vi "initalize dual gating(SubVI).vi"(0 "簇":T1={"initialize"=enum."SR830", "6221"={"6221 Resource"="GPIB0::24::INSTR", "Delta status"=FALSE, "电流|RMS(A)"=0.0}, "SR830+6221"={"source"=0, "Current(A)"=0.0, "阻抗(Ohm)"=0.0, "SR830 1"=FALSE, "SR830 2"=FALSE, "SR830 3"=FALSE, "SR830 4"=FALSE, "VISA 1"="", "VISA 2"="", "VISA 3"="", "VISA 4"="", "Reserve 1"=0, "Reserve 2"=-1, "Reserve 3"=-1, "Reserve 4"=-1, "Sensitivity 1"=-1, "Sensitivity 2"=-1, "Sensitivity 3"=-1, "Sensitivity 4"=-1, "量程入 1"=0, "量程入 2"=0, "量程入 3"=0, "量程入 4"=0}, "2400"={"2400"=FALSE, "VISA"="", "Output Level (0)"=1e-05, "Compliance  Level (0.1)"=10.0}, "ch"={"ch"=[], "current"=[], "change?"=[], "holding current\nwhen change ch?"=FALSE}, "Instrument"={"325 Resource "="GPIB0::13::INSTR", "Input (0:A) 325"=0, "Heater Output (1:1) 325"=1, "340 Resource"="GPIB0::14::INSTR", "Input (0:A) 340"=0, "Loop (0: 1)"=0, "Input (0:B) 340"=1, "Loop (1: 1)"=0, "340 Status"=refnum, "Instrument Type"=enum."PPMS-Rotate", "quantum design"=refnum, "semaphore 325"=refnum, "TCP master instance"=refnum, "M24C Resource"="GPIB0::24::INSTR", "4G supply"="GPIB0::24::INSTR", "Temp Status 24C"=refnum, "Temp"=refnum, "9T信号"=refnum, "limit"={"Field limit"=0.0, "Field rate limit"=0.0, "Temp limit"=0.0, "Temp low limit"=0.0, "Temp rate limit "=0.0}, "4g supply status"=refnum, "vi路径"="", "in-plane"="", "out-plane"="", "in-plane signal"=FALSE, "out-plane signal"=FALSE, "in plane 信号"=refnum, "pzt volt"=refnum, "Aborting"=refnum, "数据文件"=refnum, "warning"=refnum, "750 visa"="", "750 rotate"="", "335 Status 2"=refnum, "335 Resource "="GPIB0::24::INSTR", "Input (0:A) 335"=0, "Input (0:B) 335"=1, "Heater Output (1:1) 335"=1, "semaphore 340"=refnum, "semaphore 335"=refnum, "325 Status"=refnum, "semaphore 750"=refnum, "750 field status"=refnum, "camg 振荡状态"=refnum, "列表框"=refnum, "编辑列表框？"=refnum, "camg Rate"=refnum, "行数"=refnum}, "2614B"={"2614B chA"=FALSE, "2614B chB"=FALSE, "VISA"=""}, "33522b"={"33522b resource name"="GPIB0::16::INSTR", "零电压"=0.0, "最大电压"=148.0, "间隔"=4.0, "最小电压"=-48.0, "PZT Scan?"=FALSE}, "gating type"=enum."2614(daul)", "层数"=0, "行数"=0, "是否处理"=[]} {"Instrument"."Loop (1: 1)" items=["1"=1, "2"=2]; "Instrument"."Loop (0: 1)" items=["1"=1, "2"=2]; "Instrument"."Input (0:B) 340" items=["A", "B", "C", "D"]; "Instrument"."Heater Output (1:1) 335" items=["1"=1, "2"=2]; "Instrument"."Input (0:B) 335" items=["A", "B"]; "Instrument"."Input (0:A) 335" items=["A", "B"]; "Instrument"."Heater Output (1:1) 325" items=["1"=1, "2"=2]; "Instrument"."Input (0:A) 325" items=["A", "B"]; "Instrument"."Input (0:A) 340" items=["1"=1, "2"=2]; "SR830+6221"."Sensitivity 4" items=["量程每次测量会判定", "量程不变为设定值"]; "SR830+6221"."Sensitivity 3" items=["Auto Reserve"=-1, "High Reserve"=0, "Normal"=1, "Low Noise"=2]; "SR830+6221"."Sensitivity 1" items=["Auto Reserve"=-1, "High Reserve"=0, "Normal"=1, "Low Noise"=2]; "SR830+6221"."Sensitivity 2" items=["Auto Reserve"=-1, "High Reserve"=0, "Normal"=1, "Low Noise"=2]; "SR830+6221"."Reserve 4" items=["量程每次测量会判定", "量程不变为设定值"]; "SR830+6221"."Reserve 3" items=["Auto Reserve"=-1, "High Reserve"=0, "Normal"=1, "Low Noise"=2]; "SR830+6221"."Reserve 2" items=["Auto Reserve"=-1, "High Reserve"=0, "Normal"=1, "Low Noise"=2]; "SR830+6221"."Reserve 1" items=["Auto Reserve"=-1, "High Reserve"=0, "Normal"=1, "Low Noise"=2]; "SR830+6221"."source" items=["SR830 1", "SR830 2", "SR830 3", "SR830 4"]}, 2 "字符串":string) -> (7 "输出簇":T1={"initialize"=enum."SR830", "6221"={"6221 Resource"="GPIB0::24::INSTR", "Delta status"=FALSE, "电流|RMS(A)"=0.0}, "SR830+6221"={"source"=0, "Current(A)"=0.0, "阻抗(Ohm)"=0.0, "SR830 1"=FALSE, "SR830 2"=FALSE, "SR830 3"=FALSE, "SR830 4"=FALSE, "VISA 1"="", "VISA 2"="", "VISA 3"="", "VISA 4"="", "Reserve 1"=0, "Reserve 2"=-1, "Reserve 3"=-1, "Reserve 4"=-1, "Sensitivity 1"=-1, "Sensitivity 2"=-1, "Sensitivity 3"=-1, "Sensitivity 4"=-1, "量程入 1"=0, "量程入 2"=0, "量程入 3"=0, "量程入 4"=0}, "2400"={"2400"=FALSE, "VISA"="", "Output Level (0)"=1e-05, "Compliance  Level (0.1)"=10.0}, "ch"={"ch"=[], "current"=[], "change?"=[], "holding current\nwhen change ch?"=FALSE}, "Instrument"={"325 Resource "="GPIB0::13::INSTR", "Input (0:A) 325"=0, "Heater Output (1:1) 325"=1, "340 Resource"="GPIB0::14::INSTR", "Input (0:A) 340"=0, "Loop (0: 1)"=0, "Input (0:B) 340"=1, "Loop (1: 1)"=0, "340 Status"=refnum, "Instrument Type"=enum."PPMS-Rotate", "quantum design"=refnum, "semaphore 325"=refnum, "TCP master instance"=refnum, "M24C Resource"="GPIB0::24::INSTR", "4G supply"="GPIB0::24::INSTR", "Temp Status 24C"=refnum, "Temp"=refnum, "9T信号"=refnum, "limit"={"Field limit"=0.0, "Field rate limit"=0.0, "Temp limit"=0.0, "Temp low limit"=0.0, "Temp rate limit "=0.0}, "4g supply status"=refnum, "vi路径"="", "in-plane"="", "out-plane"="", "in-plane signal"=FALSE, "out-plane signal"=FALSE, "in plane 信号"=refnum, "pzt volt"=refnum, "Aborting"=refnum, "数据文件"=refnum, "warning"=refnum, "750 visa"="", "750 rotate"="", "335 Status 2"=refnum, "335 Resource "="GPIB0::24::INSTR", "Input (0:A) 335"=0, "Input (0:B) 335"=1, "Heater Output (1:1) 335"=1, "semaphore 340"=refnum, "semaphore 335"=refnum, "325 Status"=refnum, "semaphore 750"=refnum, "750 field status"=refnum, "camg 振荡状态"=refnum, "列表框"=refnum, "编辑列表框？"=refnum, "camg Rate"=refnum, "行数"=refnum}, "2614B"={"2614B chA"=FALSE, "2614B chB"=FALSE, "VISA"=""}, "33522b"={"33522b resource name"="GPIB0::16::INSTR", "零电压"=0.0, "最大电压"=148.0, "间隔"=4.0, "最小电压"=-48.0, "PZT Scan?"=FALSE}, "gating type"=enum."2614(daul)", "层数"=0, "行数"=0, "是否处理"=[]} {"Instrument"."Loop (1: 1)" items=["1"=1, "2"=2]; "Instrument"."Loop (0: 1)" items=["1"=1, "2"=2]; "Instrument"."Input (0:B) 340" items=["A", "B", "C", "D"]; "Instrument"."Heater Output (1:1) 335" items=["1"=1, "2"=2]; "Instrument"."Input (0:B) 335" items=["A", "B"]; "Instrument"."Input (0:A) 335" items=["A", "B"]; "Instrument"."Heater Output (1:1) 325" items=["1"=1, "2"=2]; "Instrument"."Input (0:A) 325" items=["A", "B"]; "Instrument"."Input (0:A) 340" items=["1"=1, "2"=2]; "SR830+6221"."Sensitivity 4" items=["量程每次测量会判定", "量程不变为设定值"]; "SR830+6221"."Sensitivity 3" items=["Auto Reserve"=-1, "High Reserve"=0, "Normal"=1, "Low Noise"=2]; "SR830+6221"."Sensitivity 1" items=["Auto Reserve"=-1, "High Reserve"=0, "Normal"=1, "Low Noise"=2]; "SR830+6221"."Sensitivity 2" items=["Auto Reserve"=-1, "High Reserve"=0, "Normal"=1, "Low Noise"=2]; "SR830+6221"."Reserve 4" items=["量程每次测量会判定", "量程不变为设定值"]; "SR830+6221"."Reserve 3" items=["Auto Reserve"=-1, "High Reserve"=0, "Normal"=1, "Low Noise"=2]; "SR830+6221"."Reserve 2" items=["Auto Reserve"=-1, "High Reserve"=0, "Normal"=1, "Low Noise"=2]; "SR830+6221"."Reserve 1" items=["Auto Reserve"=-1, "High Reserve"=0, "Normal"=1, "Low Noise"=2]; "SR830+6221"."source" items=["SR830 1", "SR830 2", "SR830 3", "SR830 4"]})   [LabVIEW 2019, in "initialize.lvlib"]
uses:
  initialize.lvlib
  ctl/config.ctl
  <vilib>/NI/Modbus Library/API/Master/Modbus Master.lvclass
  ctl/initialize.ctl
  ctl/Instrument.ctl
  ctl/335 state.ctl
  ctl/Instrument Type.ctl
  lib/QDInstrument.dll
  ctl/limit.ctl
  ctl/9T mag field stauts.ctl
  ctl/warning.ctl
  ctl/Gating type.ctl
  lib/Keithley 2600 Series/Public/Configure/Source/Configure Source (Range).vi
  lib/Keithley 2600 Series/Public/Configure/Source/Configure Source (Limit).vi
  lib/Keithley 2600 Series/Keithley 2600 Series.lvlib
panel:
  in  "Current Limit B (0.1 A) 2":dbl=0.1
  in  "Current Limit A (0.1 A)":dbl=0.1
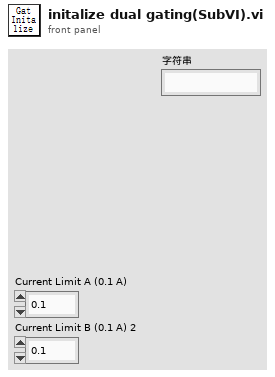
[diagram p1: front panel]
types:
  T1 = typedef "config.ctl" = cluster{"initialize":T2, "6221":cluster{"6221 Resource":refnum<visa-resource-name>, "Delta status":bool, "电流|RMS(A)":dbl}, "SR830+6221":cluster{"source":u16, "Current(A)":dbl, "阻抗(Ohm)":dbl, "SR830 1":bool, "SR830 2":bool, "SR830 3":bool, "SR830 4":bool, "VISA 1":refnum<visa-resource-name>, "VISA 2":refnum<visa-resource-name>, "VISA 3":refnum<visa-resource-name>, "VISA 4":refnum<visa-resource-name>, "Reserve 1":i16, "Reserve 2":i16, "Reserve 3":i16, "Reserve 4":i16, "Sensitivity 1":i16, "Sensitivity 2":i16, "Sensitivity 3":i16, "Sensitivity 4":i16, "量程入 1":i32, "量程入 2":i32, "量程入 3":i32, "量程入 4":i32}, "2400":cluster{"2400":bool, "VISA":refnum<visa-resource-name>, "Output Level (0)":dbl, "Compliance  Level (0.1)":dbl}, "ch":cluster{"ch":i32[], "current":dbl[], "change?":bool[], "holding current\nwhen change ch?":bool}, "Instrument":T3, "2614B":cluster{"2614B chA":bool, "2614B chB":bool, "VISA":refnum<visa-resource-name>}, "33522b":cluster{"33522b resource name":refnum<visa-resource-name>, "零电压":dbl, "最大电压":dbl, "间隔":dbl, "最小电压":dbl, "PZT Scan?":bool}, "gating type":T7, "层数":i32, "行数":i32, "是否处理":bool[]}
  T2 = typedef "initialize.ctl" = enum16{"SR830", "keithley6221-SR830", "Delta", "Delta-tunnelling", "keithley6221-2182-DC", "PZT", "4200"}
  T3 = typedef "Instrument.ctl" = cluster{"325 Resource ":refnum<visa-resource-name>, "Input (0:A) 325":u16, "Heater Output (1:1) 325":u16, "340 Resource":refnum<visa-resource-name>, "Input (0:A) 340":u16, "Loop (0: 1)":u16, "Input (0:B) 340":u16, "Loop (1: 1)":u16, "340 Status":refnum<vi>, "Instrument Type":T4, "quantum design":refnum<k24>, "semaphore 325":T5, "TCP master instance":refnum<class "Modbus Master.lvclass">, "M24C Resource":refnum<visa-resource-name>, "4G supply":refnum<visa-resource-name>, "Temp Status 24C":refnum<vi>, "Temp":refnum<vi>, "9T信号":T5, "limit":T6, "4g supply status":refnum<vi>, "vi路径":string, "in-plane":refnum<visa-resource-name>, "out-plane":refnum<visa-resource-name>, "in-plane signal":bool, "out-plane signal":bool, "in plane 信号":T5, "pzt volt":refnum<vi>, "Aborting":refnum<vi>, "数据文件":refnum<vi>, "warning":refnum<vi>, "750 visa":refnum<visa-resource-name>, "750 rotate":refnum<visa-resource-name>, "335 Status 2":refnum<vi>, "335 Resource ":refnum<visa-resource-name>, "Input (0:A) 335":u16, "Input (0:B) 335":u16, "Heater Output (1:1) 335":u16, "semaphore 340":T5, "semaphore 335":T5, "325 Status":refnum<vi>, "semaphore 750":T5, "750 field status":refnum<vi>, "camg 振荡状态":refnum<vi>, "列表框":refnum<vi>, "编辑列表框？":refnum<vi>, "camg Rate":refnum<vi>, "行数":refnum<vi>}
  T4 = typedef "Instrument Type.ctl" = enum16{"PPMS", "VersaLab", "DynaCool", "SVSM", "PPMS-Rotate", "Lakeshore335", "lengtou2", "9T mag", "9T cmag rotate", "test"}
  T5 = typedef "Semaphore RefNum" = refnum<k1>
  T6 = typedef "limit.ctl" = cluster{"Field limit":dbl, "Field rate limit":dbl, "Temp limit":dbl, "Temp low limit":dbl, "Temp rate limit ":dbl}
  T7 = typedef "Gating type.ctl" = enum32{"null", "2614(daul)", "2400"}
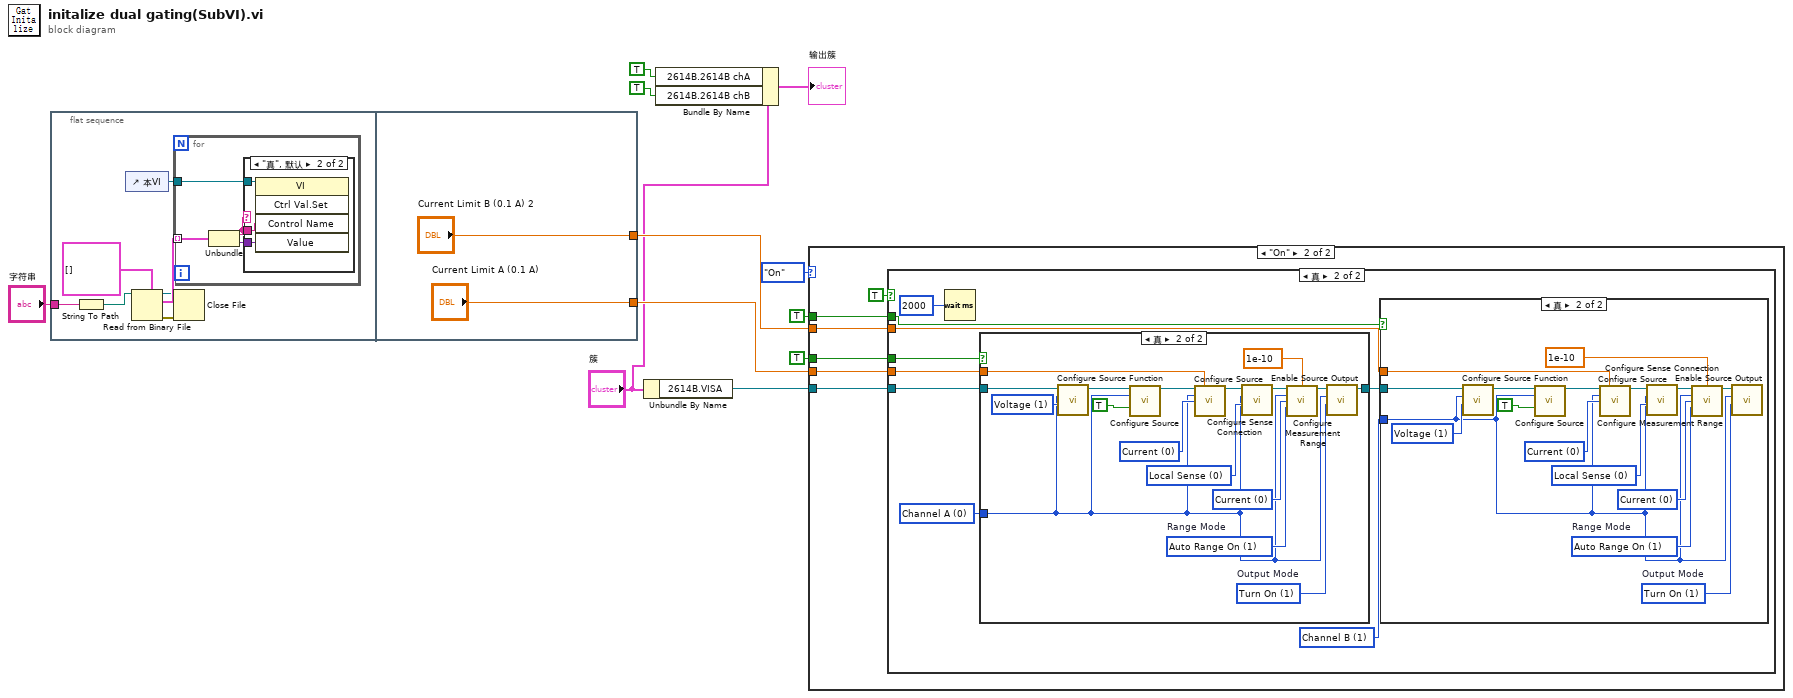
[diagram p0: block diagram]
diagram:
  n1 = flat-sequence {
    tunnel: "字符串" -> [w12]
    tunnel: ["Current Limit A (0.1 A)"] -> w8
    tunnel: ["Current Limit B (0.1 A) 2"] -> w9
    frame #0 {
      n2 = String To Path(string=w12) -> (path=w17:path)
      n3 = control-ref of="本VI"() -> (w18:refnum<vi>)
      n4 = Read from Binary File(5:cluster{"Name":string, "Variant Data":variant}[] [] ("控件值:获取全部"), 11:w17) -> (0:w13:errorcluster, 2:w15:cluster{"Name":string, "Variant Data":variant}[], 3:w14:refnum<file>)  [unwired: 4 in, 1 out]
      n5 = for {
        tunnel: w15 -> [w22] mode=indexing
        tunnel: w18 -> [w21]
        n6 = Unbundle(w22) -> ("Name"=w19:string, "Variant Data"=w20:variant)
        n7 = case shown="\"真\", 默认" w19 {
          tunnel: w21 -> [_ w25]
          tunnel: w19 -> [_ w24]
          tunnel: w20 -> [_ w23]
          frame "cancel", "load", "model", "ok" {
          }
          frame "真", Default {
            n8 = invoke class="VI" method="Ctrl Val.Set"(reference=w25, "Control Name"=w24, "Value"=w23) -> ()  [unwired: 2 in, 5 out]
          }
        }
      }
      n9 = Close File(refnum=w14, error in=w13) -> ()  [unwired: 2 out]
    }
    frame #1 {
    }
  }
  n10 = Unbundle By Name("簇") -> ("2614B.VISA"=w7:refnum<visa-resource-name>)
  n11 = Bundle By Name(cluster="簇", "2614B.2614B chA"=TRUE, "2614B.2614B chB"=TRUE) -> (→"输出簇":T1)
  n12 = case shown="\"On\"" enum16{"Off", "On"}."On" ("Output State") {
    tunnel: TRUE ("chB") -> [_ w32]
    tunnel: w9 -> [_ w31]
    tunnel: TRUE ("chA") -> [_ w30]
    tunnel: w7 -> [_ w29]
    tunnel: w8 -> [_ w28]
    frame "Off", Default {
    }
    frame "On" {
      n13 = case shown="真" TRUE {
        tunnel: w32 -> [_ w40]
        tunnel: w31 -> [_ w38]
        tunnel: w30 -> [_ w37]
        tunnel: w29 -> [_ w36]
        tunnel: w28 -> [_ w34]
        frame False {
        }
        frame True {
          w35 = 0 items=["Channel A", "Channel B"] ("Source Measure Unit Channel (0: Channel A)")
          w39 = 1 items=["Channel A", "Channel B"] ("Source Measure Unit Channel (0: Channel A)")
          n14 = Wait (ms)(milliseconds to wait=u32 2000) -> ()  [unwired: 1 out]
          n15 = case shown="真" w37 {
            tunnel: w36 -> [w59 w66]
            tunnel: w35 -> [_ w65]
            tunnel: w34 -> [_ w63]
            tunnel: [w59 w61] -> w41
            frame False {
            }
            frame True {
              w72 = 0 items=["Local Sense", "Remote Sense"] ("Sense Mode (0: Local Sense)")
              w71 = 0 items=["Current", "Voltage"] ("Range Type (0: Current)")
              w69 = 0 items=["Current", "Voltage", "Power"] ("Limit Type (1: Voltage)")
              w67 = 1 items=["Current", "Voltage"] ("Source Function (1: Voltage)")
              w70 = 1 items=["Auto Range Off", "Auto Range On", "Auto Range Follow Limit"]  # Range Mode
              w73 = 1 items=["Turn off", "Turn On", "High-Z"]  # Output Mode
              n16 = call "Configure Source Function.vi"("Source Function (1: Voltage)"=w67, "Source Measure Unit Channel (0: Channel A)"=w65, "VISA resource name"=w66) -> ("VISA resource name out"=w74:refnum<visa-resource-name>)  [unwired: 7 in, 1 out]
              n17 = call-poly "Configure Source.vi"("VISA resource name"=w74, "Source Measure Unit Channel (0: Channel A)"=w65, "Auto Range (T: Enable)"=TRUE) -> ("VISA resource name out"=w75:refnum<visa-resource-name>)  [unwired: 11 in, 1 out]
              n18 = call-poly "Configure Source.vi"("VISA resource name"=w75, "Current Limit (0.1 A)"=w63, "Source Measure Unit Channel (0: Channel A)"=w65, "Limit Type (1: Voltage)"=w69) -> ("VISA resource name out"=w76:refnum<visa-resource-name>)  [unwired: 10 in, 1 out]
              n19 = call "Configure Sense Connection.vi"("Sense Mode (0: Local Sense)"=w72, "Source Measure Unit Channel (0: Channel A)"=w65, "VISA resource name"=w76) -> ("VISA resource name out"=w64:refnum<visa-resource-name>)  [unwired: 7 in, 1 out]
              n20 = call "Configure Measurement Range.vi"("VISA resource name"=w64, "Minimum Current Range (0.1 A)"=1e-10, "Source Measure Unit Channel (0: Channel A)"=w65, "Range Type (0: Current)"=w71, "Range Mode (1: Auto Range On)"=w70) -> ("VISA resource name out"=w62:refnum<visa-resource-name>)  [unwired: 9 in, 1 out]
              n21 = call "Enable Source Output.vi"("Output Mode (0: Turn off)"=w73, "Source Measure Unit Channel (0: Channel A)"=w65, "VISA resource name"=w62) -> ("VISA resource name out"=w61:refnum<visa-resource-name>)  [unwired: 7 in, 1 out]
            }
          }
          n22 = case shown="真" w40 {
            tunnel: w41 -> [_ w48]
            tunnel: w39 -> [_ w47]
            tunnel: w38 -> [_ w45]
            frame False {
            }
            frame True {
              w54 = 0 items=["Local Sense", "Remote Sense"] ("Sense Mode (0: Local Sense)")
              w53 = 0 items=["Current", "Voltage"] ("Range Type (0: Current)")
              w51 = 0 items=["Current", "Voltage", "Power"] ("Limit Type (1: Voltage)")
              w49 = 1 items=["Current", "Voltage"] ("Source Function (1: Voltage)")
              w52 = 1 items=["Auto Range Off", "Auto Range On", "Auto Range Follow Limit"]  # Range Mode
              w55 = 1 items=["Turn off", "Turn On", "High-Z"]  # Output Mode
              n23 = call "Configure Source Function.vi"("Source Function (1: Voltage)"=w49, "Source Measure Unit Channel (0: Channel A)"=w47, "VISA resource name"=w48) -> ("VISA resource name out"=w56:refnum<visa-resource-name>)  [unwired: 7 in, 1 out]
              n24 = call-poly "Configure Source.vi"("VISA resource name"=w56, "Source Measure Unit Channel (0: Channel A)"=w47, "Auto Range (T: Enable)"=TRUE) -> ("VISA resource name out"=w57:refnum<visa-resource-name>)  [unwired: 11 in, 1 out]
              n25 = call-poly "Configure Source.vi"("VISA resource name"=w57, "Current Limit (0.1 A)"=w45, "Source Measure Unit Channel (0: Channel A)"=w47, "Limit Type (1: Voltage)"=w51) -> ("VISA resource name out"=w58:refnum<visa-resource-name>)  [unwired: 10 in, 1 out]
              n26 = call "Configure Sense Connection.vi"("Sense Mode (0: Local Sense)"=w54, "Source Measure Unit Channel (0: Channel A)"=w47, "VISA resource name"=w58) -> ("VISA resource name out"=w46:refnum<visa-resource-name>)  [unwired: 7 in, 1 out]
              n27 = call "Configure Measurement Range.vi"("VISA resource name"=w46, "Minimum Current Range (0.1 A)"=1e-10, "Source Measure Unit Channel (0: Channel A)"=w47, "Range Type (0: Current)"=w53, "Range Mode (1: Auto Range On)"=w52) -> ("VISA resource name out"=w44:refnum<visa-resource-name>)  [unwired: 9 in, 1 out]
              n28 = call "Enable Source Output.vi"("Output Mode (0: Turn off)"=w55, "Source Measure Unit Channel (0: Channel A)"=w47, "VISA resource name"=w44) -> ()  [unwired: 7 in, 2 out]
            }
          }
        }
      }
    }
  }
